vi "Read Unique Test ID.vi"(11 "Test Assert in":refnum<class "Test Assert.lvclass">) -> (2 "Unique Test ID":string, 3 "Test Assert out":refnum<class "Test Assert.lvclass">)   [LabVIEW 2013, in "Caraya.lvlib" / "Test Assert.lvclass"]
uses:
  Test Assert.lvclass
  Test Assert.lvclass/Test Assert.ctl
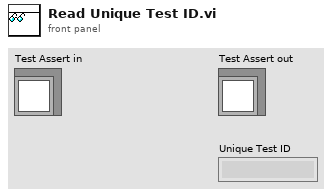
[diagram p1: front panel]
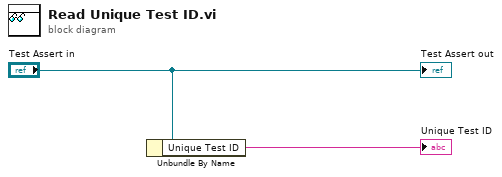
[diagram p0: block diagram]
diagram:
  n1 = Unbundle By Name("Test Assert in") -> ("Unique Test ID"=→"Unique Test ID":string)
  "Test Assert out" <- "Test Assert in"
